vi "Time Info.vi"(11 "测试人":string="User 1") -> (0 "字符串":string, 1 "测试者":string="User 1", 2 "日期":string="2007-9-9", 3 "时间":string="2:54")   [LabVIEW 2014]
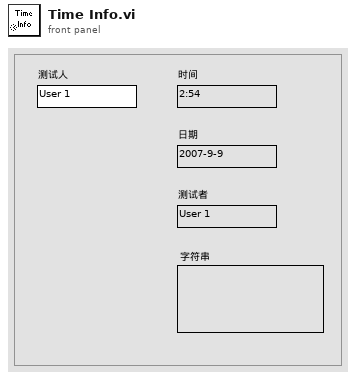
[diagram p1: front panel]
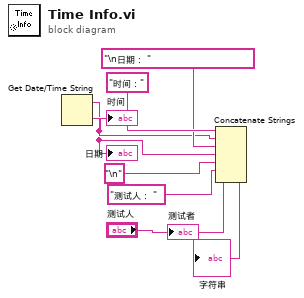
[diagram p0: block diagram]
diagram:
  n1 = Get Date/Time String() -> (date string=w1:string, time string=w2:string)  [unwired: 3 in]
  "日期" <- w1
  "时间" <- w2
  n2 = Concatenate Strings("时间：" ("Substring"), w2, "\n日期： " ("Substring"), w1, "\n" ("Substring"), "测试人： " ("Substring"), "测试人") -> (→"字符串":string)
  "测试者" <- "测试人"
